vi "UE9 Single IO Example.vi"() -> (0 "error out":errorcluster)   [LabVIEW 2021]
panel:
  in  "IOType Ring":u16(ring) items=["LJ_ioGET_AIN", "LJ_ioPUT_DAC", "LJ_ioGET_DIGITAL_BIT", "LJ_ioGET_DIGITAL_PORT", "LJ_ioPUT_DIGITAL_BIT", "LJ_ioPUT_DIGITAL_PORT", "LJ_ioGET_COUNTER", "LJ_ioGET_TIMER"]
  in  "x1":i32
  in  "FirstFound":bool=TRUE
  in  "ConnectionType":u16(ring) items=["LJ_ctUSB", "LJ_ctETHERNET"]
  in  "Address":string="192.168.1.209"
  in  "Value Write":dbl format="%.3f"
  out "Error Message":string
  out "Value Read":dbl format="%.6f"
  in  "Channel #":i32
  # "Reads 1 input or writes 1 output.  Does not do any configuration (such as resolution\nor range for analog inputs)."
  # "Specify an IP address for Ethernet, or Local ID\nfor USB.  If FirstFound is selected, Local ID is\nignored for USB."
  # "Used for digital port IOtypes where\nx1 specifies the # of bits and then\nChannel # specifies starting channel.\nFor differential AIN, x1 specifies\nnegative channel."
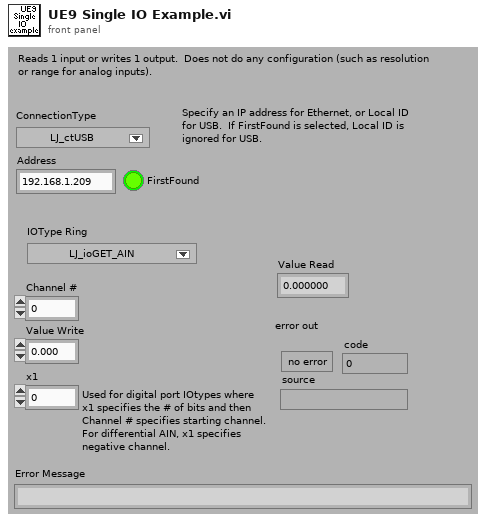
[diagram p1: front panel]
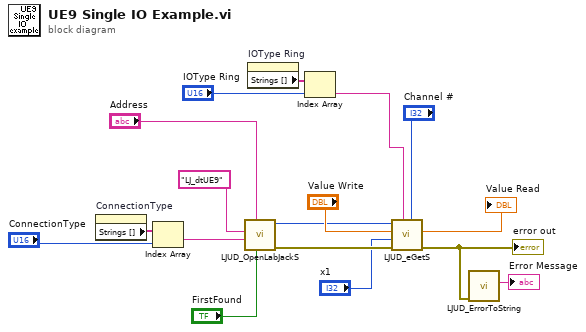
[diagram p0: block diagram]
diagram:
  n1 = property on="ConnectionType" class="Ring (strict)"() -> ("Strings []"=w6:string[])  [unwired: 2 in, 2 out]
  n2 = Index Array(array=w6, index="ConnectionType") -> (element=w5:string)
  n3 = call "LJUD_OpenLabJackS.vi"("FirstFound"="FirstFound", "Address"="Address", "ConnectionType"=w5, "DeviceType"="LJ_dtUE9") -> ("error out"=w13:errorcluster, "Handle"=w8:i32)  [unwired: 5 in, 1 out]
  n4 = property on="IOType Ring" class="Ring (strict)"() -> ("Strings []"=w4:string[])  [unwired: 2 in, 2 out]
  n5 = Index Array(array=w4, index="IOType Ring") -> (element=w2:string)
  n6 = call "LJUD_eGetS.vi"("Channel"="Channel #", "IOType"=w2, "error in"=w13, "x1"="x1", "Value Write"="Value Write", "Handle In"=w8) -> ("error out"=w14:errorcluster, "Value Read"=→"Value Read":dbl)  [unwired: 3 in, 1 out]
  "error out" <- w14
  n7 = call "LJUD_ErrorToString.vi"("error in"=w14) -> ("String"=→"Error Message":string)  [unwired: 10 in]
